vi "SHAPE_FitnessFunction.vi"(1 "Init? (F)":bool, 2 "Data":variant, 3 "Phenotype":i32[](array[numeric])) -> (0 "Fitness":dbl)   [LabVIEW 2016, in "Shapelets Search (GA).lvlib"]
uses:
  Shapelets Search (GA).lvlib
  Shapelets Search GA.lvclass
panel:
  # "This VI is a part of BCI Design library, http://www.ru-bci.org \nCopyright © 2020, Sotnikov Peter, All rights reserved. License: CC BY-NC 4.0"
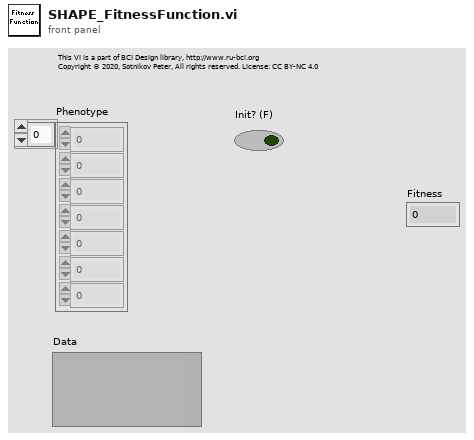
[diagram p1: front panel]
types:
  T1 = typedef "Shapelets Search (GA).lvlib/SHAPE_SearchTypes.ctl" = enum16{"Лучший шейплет", "Набор шейплетов"}
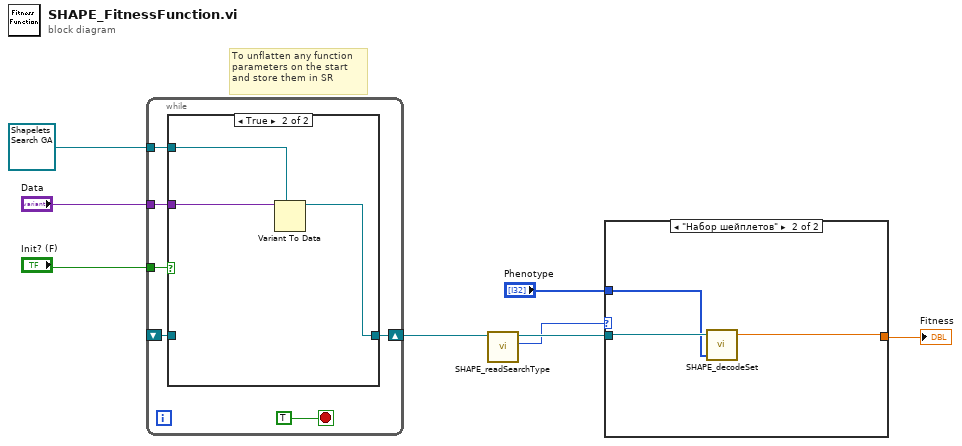
[diagram p0: block diagram]
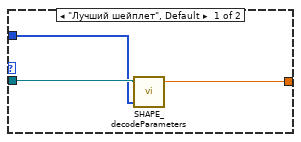
[diagram p2: hidden frame]
diagram:
  # "To unflatten any function\nparameters on the start\nand store them in SR"
  n1 = while {
    tunnel: "Data" -> [w12]
    tunnel: "Init? (F)" -> [w13]
    shift-right: [w11] -> w2
    shift-left: _ -> [w10]
    tunnel: refnum<class "Shapelets Search GA.lvclass"> refnum ("Shapelets Search (GA).lvlib:Shapelets Search GA.lvclass") -> [w9]
    stop <- TRUE stop-if-true
    n2 = case shown="True" w13 {
      tunnel: w12 -> [_ w18]
      tunnel: [w15 w17] -> w11
      tunnel: w10 -> [w15 _]
      tunnel: w9 -> [_ w16]
      frame False {
      }
      frame True {
        n3 = Variant To Data(type=w16, Variant=w18) -> (data=w17:refnum<class "Shapelets Search GA.lvclass">)  [unwired: 1 in, 1 out]
      }
    }
  }
  n4 = call-dynamic "SHAPE_readSearchType.vi"("BandGlobalOpt in"=w2) -> ("ClassifierTypes"=w3:T1, "BandGlobalOpt out"=w6:refnum<class "Shapelets Search GA.lvclass">)  [unwired: 8 in, 1 out]
  n5 = case shown="\"Набор шейплетов\"" w3 {
    tunnel: w6 -> [w21 w24]
    tunnel: "Phenotype" -> [w20 w22]
    tunnel: [w19 w23] -> w4
    frame "Лучший шейплет", Default {
      n6 = call "SHAPE_decodeParameters.vi"("Parameters"=w20, "BandGlobalOpt.lvclass"=w21) -> ("Accuracy"=w19:sgl)  [unwired: 2 in, 1 out]
    }
    frame "Набор шейплетов" {
      n7 = call "SHAPE_decodeSet.vi"("Parameters"=w22, "BandGlobalOpt.lvclass"=w24) -> ("Accuracy"=w23:sgl)  [unwired: 3 in]
    }
  }
  "Fitness" <- w4
